vi "Key-Value To Packet Data.vi"(9 "Value":variant, 10 "Key":variant) -> (1 "Packet":T1, 2 "Packed String":string)   [LabVIEW 2018, in "Application.lvlib" / "Store.lvclass"]
uses:
  Store.lvclass
  Controls/Packet.ctl
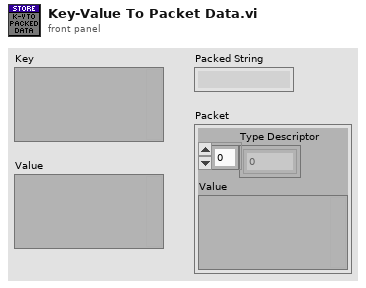
[diagram p1: front panel]
types:
  T1 = typedef "Application.lvlib/Store.lvclass/Packet.ctl" = cluster{"Type Descriptor":i16[], "Value":variant}
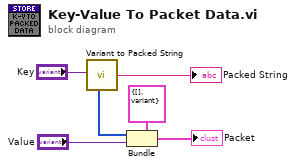
[diagram p0: block diagram]
diagram:
  n1 = call "Variant to Packed String.vi"("Variant"="Key") -> ("Type Descriptor"=w3:i16[], "Packed String"=→"Packed String":string)  [unwired: 3 in]
  n2 = Bundle(cluster=T1 {"Type Descriptor"=[], "Value"=variant} ("Packet"), "Type Descriptor"=w3, "Value"="Value") -> (→"Packet":T1)
